vi "Handle setConfiguration.vi"(8 "error in (no error)":errorcluster, 10 "setConfiguration":variant, 11 "Instrument.FrameworkTemplate":refnum<class "Instrument.Temperhum.lvclass">) -> (0 "error out":errorcluster, 3 "Instrument.FrameworkTemplate out":refnum<class "Instrument.Temperhum.lvclass">)   [LabVIEW 2019, in "Instrument.Temperhum.lvclass"]
uses:
  Instrument.Temperhum.lvclass
  Instrument.Temperhum.lvclass/Instrument.Temperhum.ctl
  7fd627c4-46b3-46d4-9a3c-07d9147c5e06.vi
  7fd627c4-46b3-46d4-9a3c-07d9147c5e06.vi/3de891d5-ce89-4d18-8dc3-42f1f2bfe5f8.vi
  7fd627c4-46b3-46d4-9a3c-07d9147c5e06.vi/4e208e92-295e-4d0d-86fa-250aead57436.vi
  <vilib>/Utility/Data Type/Get Type Information.vi
  <vilib>/JDP Science/JSONtext/JSON text to Variant.vi
  <vilib>/JDP Science/JSONtext/LVClass Serializer/JSONtext LVClass Serializer.lvclass
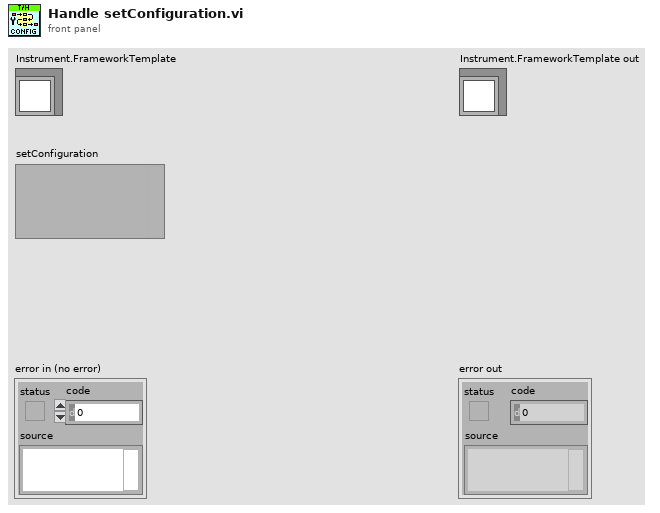
[diagram p1: front panel]
types:
  T1 = typedef "Instrument.Temperhum.lvclass/Instrument.Temperhum.Configuration--Cluster.ctl" = cluster{"Example Setting 1":dbl, "Example Setting 2":dbl, "Logpath":string}
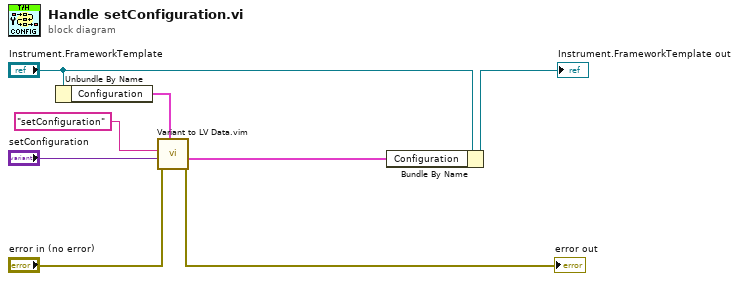
[diagram p0: block diagram]
diagram:
  n1 = Unbundle By Name("Instrument.FrameworkTemplate") -> ("Configuration"=w7:T1)
  n2 = call "Variant to LV Data.vim"("type"=w7, "error in (no error)"="error in (no error)", "JSON Data in"="setConfiguration", "Command"="setConfiguration") -> ("error out"=→"error out":errorcluster, "Data out"=w1:T1)  [unwired: 4 in, 2 out]
  n3 = Bundle By Name(cluster="Instrument.FrameworkTemplate", "Configuration"=w1) -> (→"Instrument.FrameworkTemplate out":refnum<class "Instrument.Temperhum.lvclass">)
